vi "Modulator.vi"(0 "Sampling frequency":dbl, 1 "Modulation Type":T1=enum."Simple", 2 "Input Signal":dbl[](array[numeric]), 3 "Carrier Frequency":dbl=40000.0, 5 "Modulation depth":dbl=0.8) -> (7 "Output signal":dbl[](array[numeric]))   [LabVIEW 2016]
uses:
  Modulation_types.ctl
  <vilib>/Analysis/NI_AALBase.lvlib
  <vilib>/Analysis/NI_AALPro.lvlib
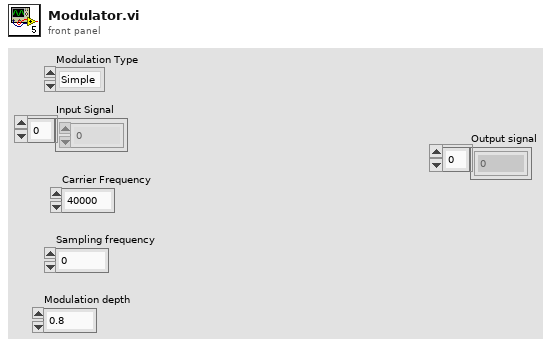
[diagram p1: front panel]
types:
  T1 = typedef "Modulation_types.ctl" = enum16{"None", "Add", "Simple", "Offset", "Square root", "Exponential"}
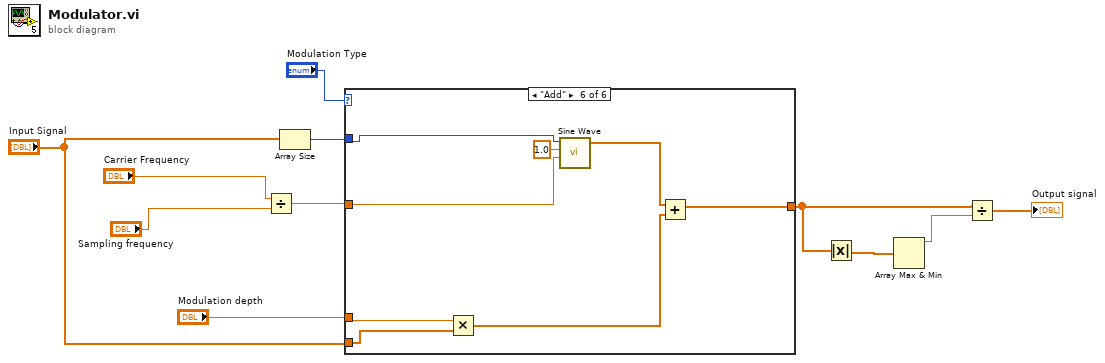
[diagram p0: block diagram]
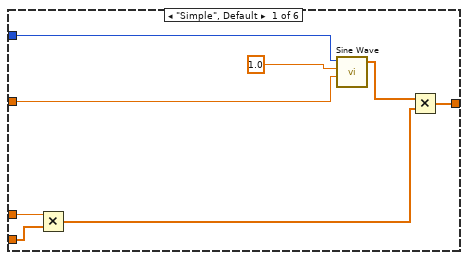
[diagram p2: hidden frame]
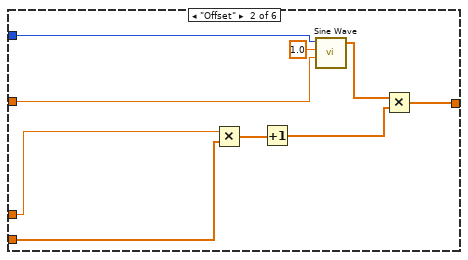
[diagram p3: hidden frame]
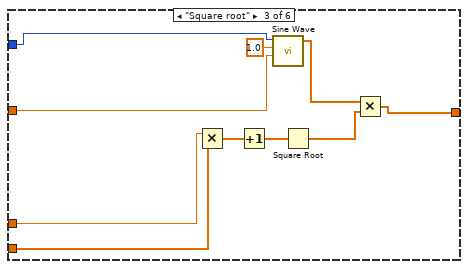
[diagram p4: hidden frame]
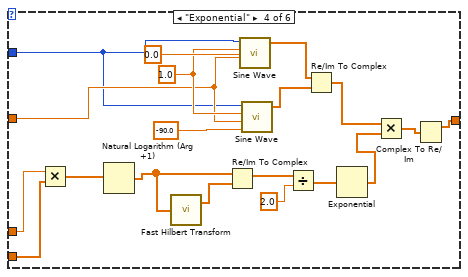
[diagram p5: hidden frame]
diagram:
  n1 = Divide(x="Carrier Frequency", y="Sampling frequency") -> (x/y=w7:dbl)
  n2 = Array Size(array="Input Signal") -> (size(s)=w10:i32)
  n3 = case shown="\"Add\"" "Modulation Type" {
    tunnel: [w16 w24 w33 w44 w58 w59] -> w2
    tunnel: w10 -> [w15 w20 w29 w39 _ w64]
    tunnel: w7 -> [w14 w21 w30 w40 _ w65]
    tunnel: "Modulation depth" -> [w13 w23 w32 w43 _ w63]
    tunnel: "Input Signal" -> [w12 w22 w31 w42 w58 w62]
    frame "Simple", Default {
      n4 = Multiply(x=w13, y=w12) -> (x*y=w17:dbl[])
      n5 = call <vilib>:"Sine Wave.vi"("samples"=w15, "amplitude"=1.0, "frequency"=w14) -> ("sine wave"=w18:dbl[])  [unwired: 2 in, 2 out]
      n6 = Multiply(x=w18, y=w17) -> (x*y=w16:dbl[])
    }
    frame "Offset" {
      n7 = Multiply(x=w23, y=w22) -> (x*y=w27:dbl[])
      n8 = Increment(x=w27) -> (x+1=w25:dbl[])
      n9 = call <vilib>:"Sine Wave.vi"("samples"=w20, "amplitude"=1.0, "frequency"=w21) -> ("sine wave"=w26:dbl[])  [unwired: 2 in, 2 out]
      n10 = Multiply(x=w26, y=w25) -> (x*y=w24:dbl[])
    }
    frame "Square root" {
      n11 = Multiply(x=w32, y=w31) -> (x*y=w37:dbl[])
      n12 = Increment(x=w37) -> (x+1=w36:dbl[])
      n13 = call <vilib>:"Sine Wave.vi"("samples"=w29, "amplitude"=1.0, "frequency"=w30) -> ("sine wave"=w35:dbl[])  [unwired: 2 in, 2 out]
      n14 = Square Root(x=w36) -> (sqrt(x)=w34:dbl[])
      n15 = Multiply(x=w35, y=w34) -> (x*y=w33:dbl[])
    }
    frame "Exponential" {
      w55 = 1.0 ("amplitude")
      n16 = Multiply(x=w43, y=w42) -> (x*y=w52:dbl[])
      n17 = Natural Logarithm (Arg +1)(1:w52) -> (0:w41:dbl[])
      n18 = call <vilib>:"Fast Hilbert Transform.vi"("X"=w41) -> ("Hilbert{X}"=w51:dbl[])  [unwired: 1 out]
      n19 = Re/Im To Complex(1:w51, 2:w41) -> (0:w49:cdb[])
      n20 = call <vilib>:"Sine Wave.vi"("samples"=w39, "amplitude"=w55, "frequency"=w40, "phase in"=0.0) -> ("sine wave"=w54:dbl[])  [unwired: 1 in, 2 out]
      n21 = call <vilib>:"Sine Wave.vi"("samples"=w39, "amplitude"=w55, "frequency"=w40, "phase in"=-90.0) -> ("sine wave"=w53:dbl[])  [unwired: 1 in, 2 out]
      n22 = Divide(x=w49, y=2.0) -> (x/y=w46:cdb[])
      n23 = Re/Im To Complex(1:w53, 2:w54) -> (0:w48:cdb[])
      n24 = Exponential(1:w46) -> (0:w47:cdb[])
      n25 = Multiply(x=w48, y=w47) -> (x*y=w45:cdb[])
      n26 = Complex To Re/Im(x + iy=w45) -> (x=w44:dbl[])  [unwired: 1 out]
    }
    frame "None" {
    }
    frame "Add" {
      n27 = Multiply(x=w63, y=w62) -> (x*y=w61:dbl[])
      n28 = call <vilib>:"Sine Wave.vi"("samples"=w64, "amplitude"=1.0, "frequency"=w65) -> ("sine wave"=w60:dbl[])  [unwired: 2 in, 2 out]
      n29 = Add(x=w60, y=w61) -> (x+y=w59:dbl[])
    }
  }
  n30 = Absolute Value(x=w2) -> (abs(x)=w4:dbl[])
  n31 = Array Max & Min(array=w4) -> (max value=w3:dbl)  [unwired: 3 out]
  n32 = Divide(x=w2, y=w3) -> (x/y=→"Output signal":dbl[])
